vi "Add Timestamp Channel.vi"(8 "error in":errorcluster, 11 "message section":T1 format="%.0x") -> (0 "error out":errorcluster, 2 "timestamp channel":T1 format="%.0x", 3 "message section out":T1 format="%.0x")   [LabVIEW 2020, in "AIM MIL-STD-1553 Scripting.lvlib"]
doc: "Adds a <b>timestamp channel</b> to the specified <b>message section</b> and returns a reference to the added channel."
uses:
  AIM MIL-STD-1553 Scripting.lvlib
  <vilib>/NI VeriStand/Custom Device API/Custom Device Item Ref.ctl
  <vilib>/NI VeriStand/Custom Device API/Custom Device Channel.ctl
  <vilib>/NI VeriStand/Custom Device API/Custom Device Channel Type.ctl
  Constants.vi
  <vilib>/NI VeriStand/Custom Device API/Custom Device API.lvlib
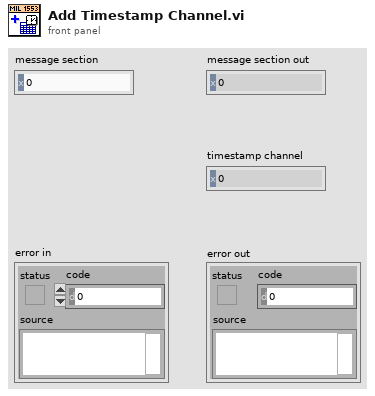
[diagram p1: front panel]
types:
  T1 = typedef "Custom Device API.lvlib/Custom Device Item Ref.ctl" = u64
  T2 = typedef "Custom Device API.lvlib/Custom Device Channel.ctl" = cluster{"Type":T3, "Units":string, "Default Value":dbl, "Faultable":bool, "Scalable":bool}
  T3 = typedef "Custom Device API.lvlib/Custom Device Channel Type.ctl" = enum16{"Input", "Output"}
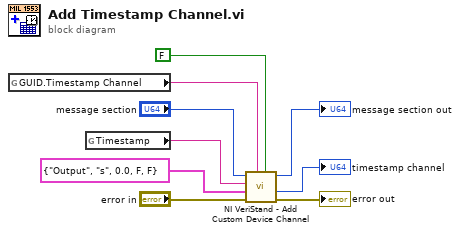
[diagram p0: block diagram]
diagram:
  n1 = global read "Constants.vi" "GUID.Timestamp Channel"() -> (w2:string)
  n2 = global read "Constants.vi" "Timestamp"() -> (w3:string)
  n3 = call <vilib>:"NI VeriStand - Add Custom Device Channel.vi"("Highlight? (F)"=FALSE, "GUID (Default Channel)"=w2, "error in (no error)"="error in", "Channel"=T2 {"Type"=enum."Output", "Units"="s", "Default Value"=0.0, "Faultable"=FALSE, "Scalable"=FALSE}, "Channel Name"=w3, "Parent Ref in"="message section") -> ("error out"=→"error out":errorcluster, "Channel Ref"=→"timestamp channel":T1, "Parent Ref out"=→"message section out":T1)  [unwired: 2 in, 1 out]
